vi "PDUJsonToString.vi"(8 "error in (no error)":errorcluster, 11 "Data Out":string) -> (0 "error out":errorcluster, 3 "PUID":string)   [LabVIEW 2015]
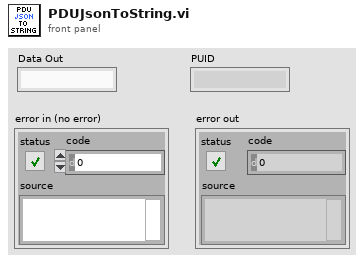
[diagram p1: front panel]
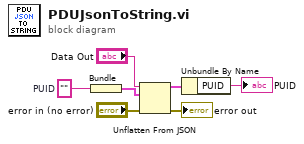
[diagram p0: block diagram]
diagram:
  w3 = ""  # PUID
  n1 = Bundle("PUID"=w3) -> (w4:cluster{"PUID":string})  [unwired: 1 in]
  n2 = Unflatten From JSON(JSON string="Data Out", type and defaults=w4, error in (no error)="error in (no error)") -> (value=w5:cluster{"PUID":string}, error out=→"error out":errorcluster)  [unwired: 4 in]
  n3 = Unbundle By Name(w5) -> ("PUID"=→"PUID":string)
